vi "Theme4_Topic4_qn21.vi"(9 "RefPrevious":refnum<vi>, 10 "RefNext":refnum<vi>, 11 "connection reference":T1) -> (2 "AnsIndicator":refnum<vi>[](array[refnum]))   [LabVIEW 2013]
uses:
  why.vi
  Precontrol.vi
  <vilib>/addons/database/Connection.llb/Conn ObjectReference.ctl
  <vilib>/addons/database/NI_Database_API.lvlib
panel:
  out "Why?":string
  out "DInd":bool
  out "CInd":bool
  out "BInd":bool
  out "AInd":bool
  in  "ABCD":enum32{"No Selection", "A", "B", "C", "D"}(radio)
  out "MCQ_Randomized":string[](array[string])
  # "An insect makes sound that is higher than the maximum audible frequency of human beings , Given that speed of sound in air is approximately 300m/s ,which of the following could be the wavelength of the sound ?"
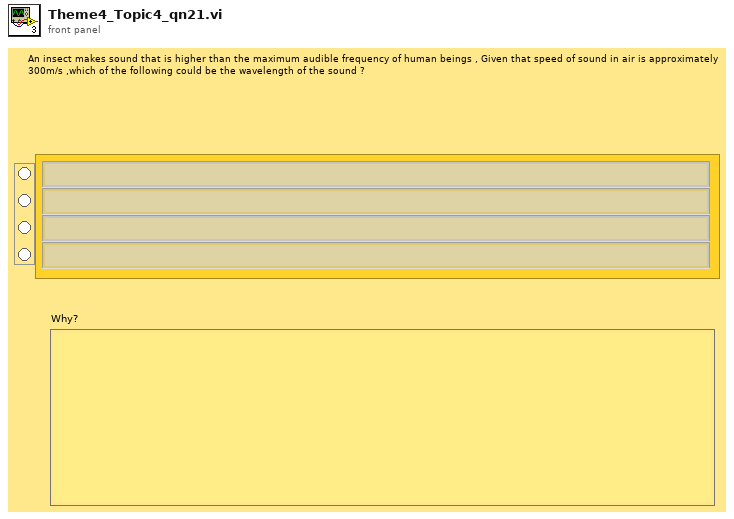
[diagram p1: front panel]
types:
  T1 = typedef "NI_Database_API.lvlib/Conn ObjectReference.ctl" = refnum<k1>
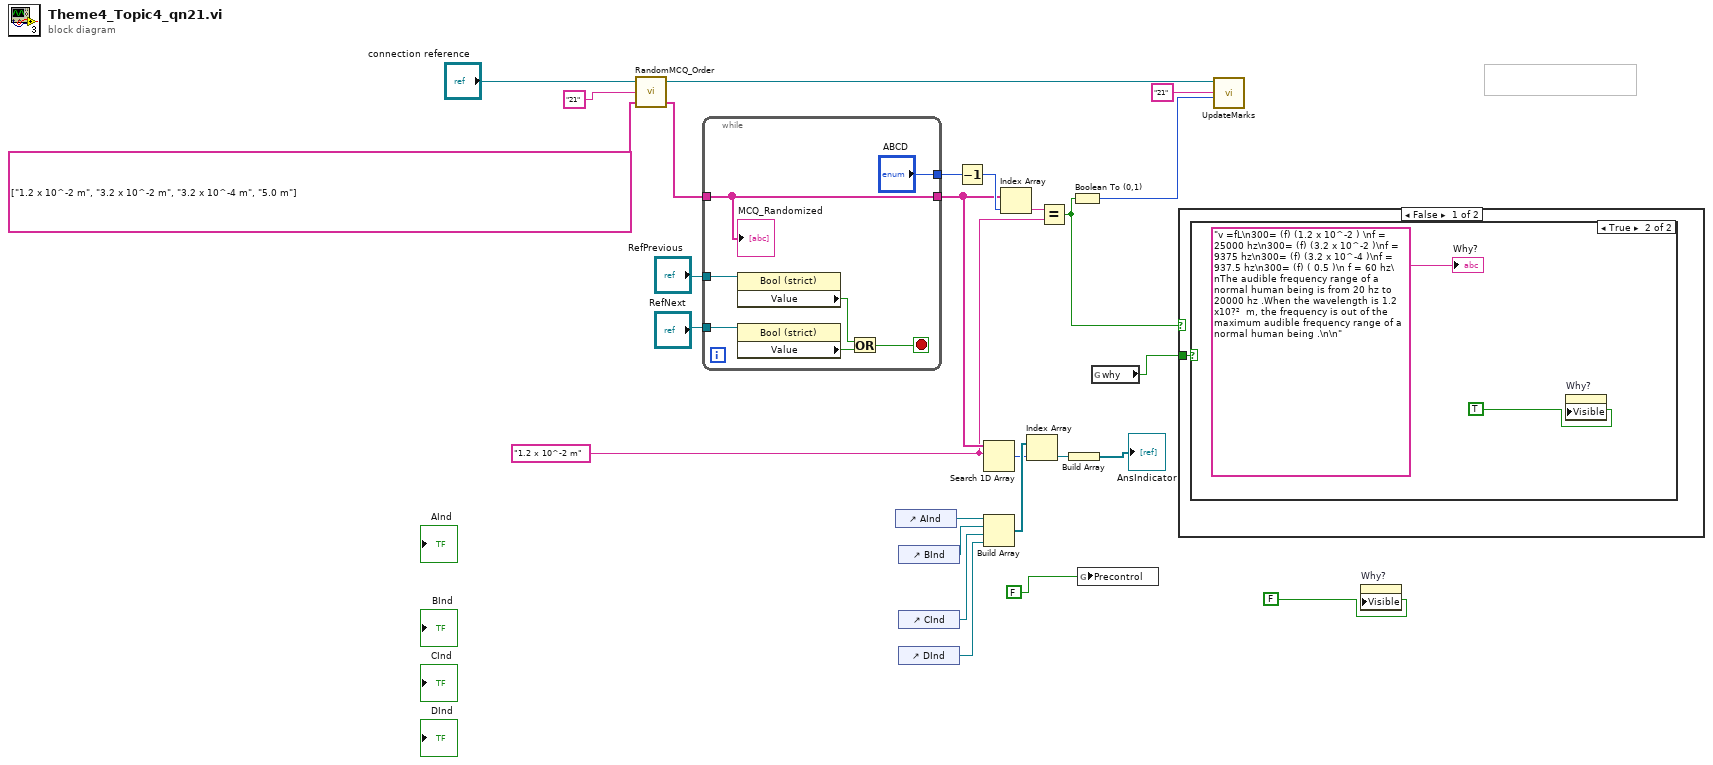
[diagram p0: block diagram]
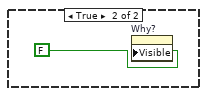
[diagram p3: hidden frame]
diagram:
  w13 = "1.2 x 10^-2 m" ("element")
  n1 = call "RandomMCQ_Order.vi"("MCQ_Ordered"=string[] ["1.2 x 10^-2 m", "3.2 x 10^-2 m", "3.2 x 10^-4 m", "5.0 m"], "Questions_Ordered"="21", "connection reference"="connection reference") -> ("MCQ_Randomized"=w26:string[], "connection reference out"=w10:T1)  [unwired: 1 in]
  n2 = while {
    tunnel: ["ABCD"] -> w2
    tunnel: w26 -> [w28]
    tunnel: [w28] -> w15
    tunnel: "RefNext" -> [w29]
    tunnel: "RefPrevious" -> [w30]
    stop <- w27 stop-if-true
    n3 = property class="Bool (strict)"(reference=w30) -> ("Value"=w32:bool)  [unwired: 1 in, 2 out]
    n4 = property class="Bool (strict)"(reference=w29) -> ("Value"=w31:bool)  [unwired: 1 in, 2 out]
    n5 = Or(x=w32, y=w31) -> (x .or. y?=w27:bool)
    "MCQ_Randomized" <- w28
  }
  n6 = control-ref of="AInd"() -> (w23:refnum<vi>)
  n7 = control-ref of="BInd"() -> (w22:refnum<vi>)
  n8 = control-ref of="CInd"() -> (w21:refnum<vi>)
  n9 = control-ref of="DInd"() -> (w20:refnum<vi>)
  n10 = Decrement(x=w2) -> (x-1=w16:enum32{"No Selection", "A", "B", "C", "D"})
  n11 = Search 1D Array(1D array=w15, element=w13) -> (index of element=w18:i32)  [unwired: 1 in]
  n12 = Build Array(w23, w22, w21, w20) -> (w19:refnum<vi>[])
  n13 = Index Array(array=w15, index=w16) -> (element=w14:string)
  n14 = Index Array(array=w19, index=w18) -> (element=w17:refnum<vi>)
  n15 = Equal?(x=w14, y=w13) -> (x = y?=w5:bool)
  n16 = Build Array(w17) -> (→"AnsIndicator":refnum<vi>[])
  n17 = Boolean To (0,1)(Boolean=w5) -> (0, 1=w6:i16)
  n18 = global write "Precontrol.vi" "Precontrol"(FALSE) -> ()
  n19 = global read "why.vi" "why"() -> (w3:bool)
  n20 = case shown="False" w5 {
    tunnel: w3 -> [w34 _]
    frame False {
      n21 = case shown="True" w34 {
        frame False {
        }
        frame True {
          n22 = property on="Why?" class="Str"("Visible"=TRUE) -> ()  [unwired: 2 in, 2 out]
          "Why?" <- "v =fL\n300= (f) (1.2 x 10^-2 ) \nf = 25000 hz\n300= (f) (3.2 x 10^-2 )\nf = 9375 hz\n300= (f) (3.2 x 10^-4 )\nf = 937.5 hz\n300= (f) ( 0.5 )\n f = 60 hz\nThe audible frequency range of a normal human being is from 20 hz to 20000 hz .When the wavelength is 1.2 x10?²  m, the frequency is out of the maximum audible frequency range of a normal human being .\n\n"
        }
      }
    }
    frame True {
      n23 = property on="Why?" class="Str"("Visible"=FALSE) -> ()  [unwired: 2 in, 2 out]
    }
  }
  n24 = call "UpdateMarks.vi"("MarksEarned"=w6, "QuestionsNo_Ordered"="21", "connection reference"=w10) -> ()  [unwired: 9 in]
  n25 = property on="Why?" class="Str"("Visible"=FALSE) -> ()  [unwired: 2 in, 2 out]
